vi "Load Becker-Hickl File.vi"(8 "Error In":errorcluster, 11 "File Path Control":path) -> (0 "Error Out":errorcluster, 1 "Measurement Information":T1 {"Measurement FCS Info"."FCS Type" format="%.0b"; "Measurement FCS Info"."FCS Decay Calc" format="%016b"; "Measurement Stop Info"."Flags" format="%016b"}, 2 "Data":sgl[][][](array[numeric]), 4 "TAC Parameters":T5 {"Frequency (Hz)" format="%#.6g"; "TAC Range (s)" format="%.6g"; "TAC Bin (s)" format="%#.6g"}, 5 "Size (in Bytes)":i64, 7 "Load Time (s)":dbl)   [LabVIEW 2021, in "Becker-Hickl Files.lvlib"]
uses:
  Becker-Hickl Files.lvlib
  Time/Time.lvlib
  Becker-Hickl Image Parameters.ctl
  Becker-Hickl TAC Parameters.ctl
  Becker-Hickl Measurement Stop Info.ctl
  Becker-Hickl FCS Measurement Info.ctl
  Becker-Hickl Additional Histogram Measurement Info.ctl
  Becker-Hickl Measurement Information.ctl
  Becker-Hickl File Header Structure.ctl
panel:
  out "Image Parameters":T6
  out "B& H File Header":T7 {"Header Valid" format="%.0x"; "# Data Blocks" format="%.0x"; "Revision" format="%.0b"}
  out "Information String":string
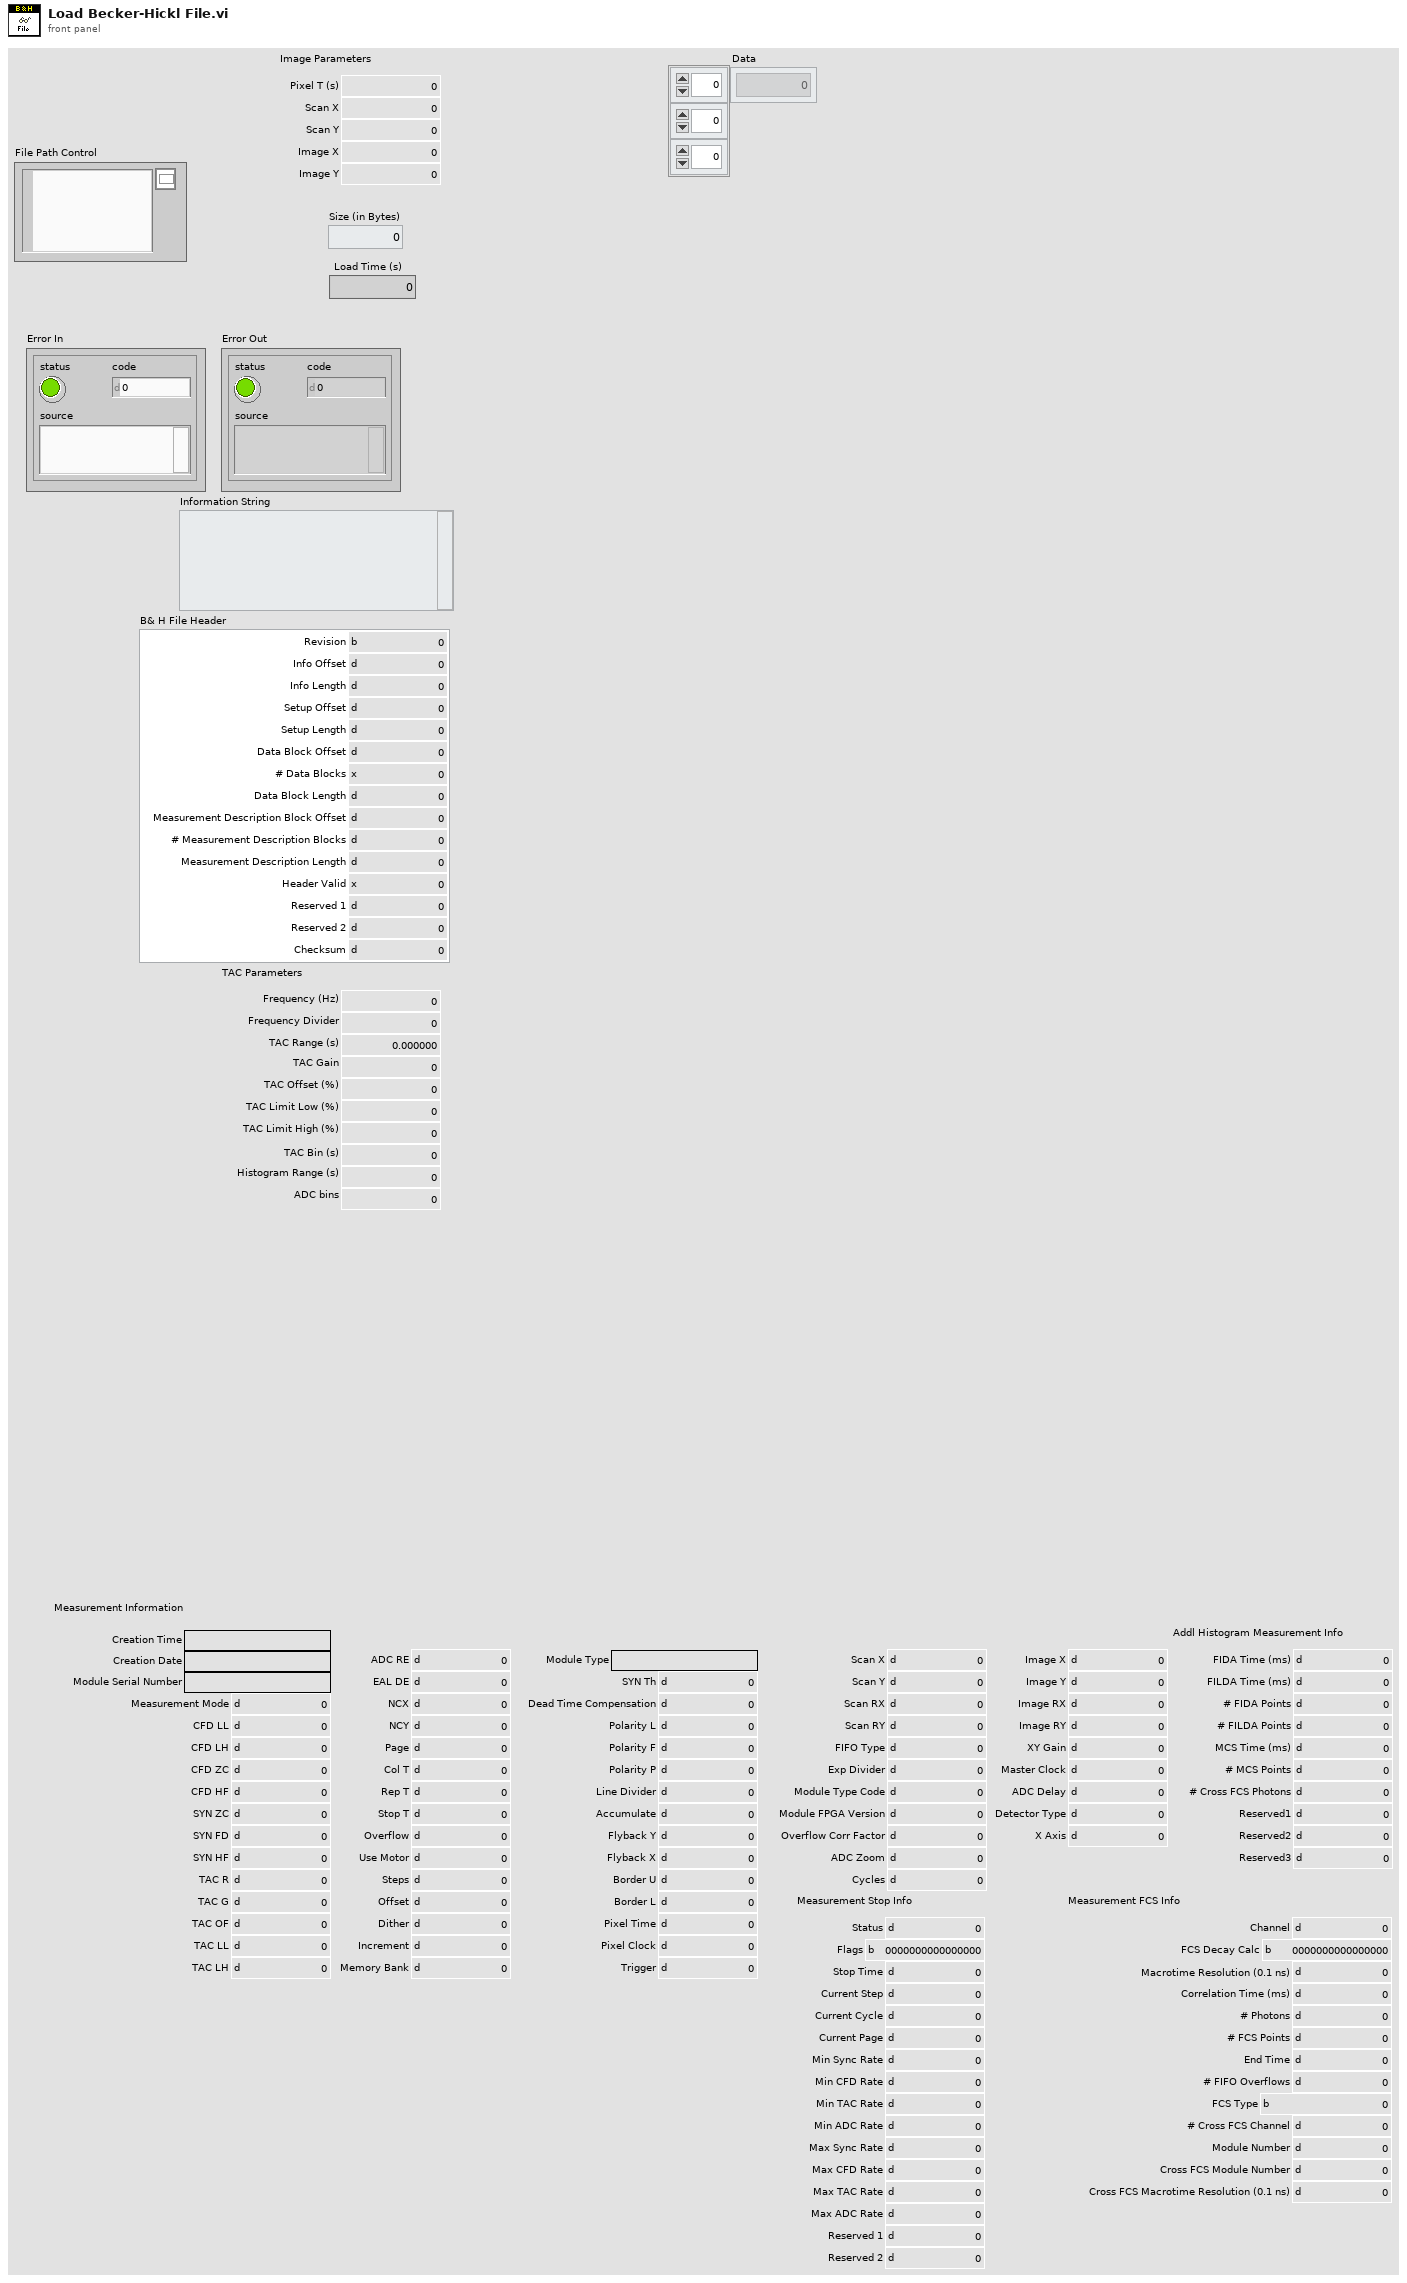
[diagram p1: front panel]
types:
  T1 = typedef "Becker-Hickl Files.lvlib/Becker-Hickl Measurement Information.ctl" = cluster{"Measurement Stop Info":T2, "Measurement FCS Info":T3, "Addl Histogram Measurement Info":T4, "Creation Time":string, "Creation Date":string, "Module Serial Number":string, "Measurement Mode":i16, "CFD LL":sgl, "CFD LH":sgl, "CFD ZC":sgl, "CFD HF":sgl, "SYN ZC":sgl, "SYN FD":i16, "SYN HF":sgl, "TAC R":sgl, "TAC G":i16, "TAC OF":sgl, "TAC LL":sgl, "TAC LH":sgl, "ADC RE":i16, "EAL DE":i16, "NCX":i16, "NCY":i16, "Page":u16, "Col T":sgl, "Rep T":sgl, "Stop T":i16, "Overflow":u8, "Use Motor":i16, "Steps":u16, "Offset":sgl, "Dither":i16, "Increment":i16, "Memory Bank":i16, "Module Type":string, "SYN Th":sgl, "Dead Time Compensation":i16, "Polarity L":i16, "Polarity F":i16, "Polarity P":i16, "Line Divider":i16, "Accumulate":i16, "Flyback Y":i32, "Flyback X":i32, "Border U":i32, "Border L":i32, "Pixel Time":sgl, "Pixel Clock":i16, "Trigger":i16, "Scan X":i32, "Scan Y":i32, "Scan RX":i32, "Scan RY":i32, "FIFO Type":i16, "Exp Divider":i32, "Module Type Code":u16, "Module FPGA Version":u16, "Overflow Corr Factor":sgl, "ADC Zoom":i32, "Cycles":i32, "Image X":i32, "Image Y":i32, "Image RX":i32, "Image RY":i32, "XY Gain":i16, "Master Clock":i16, "ADC Delay":i16, "Detector Type":i16, "X Axis":i16}
  T2 = typedef "Becker-Hickl Files.lvlib/Becker-Hickl Measurement Stop Info.ctl" = cluster{"Status":u16, "Flags":u16, "Stop Time":sgl, "Current Step":i32, "Current Cycle":i32, "Current Page":i32, "Min Sync Rate":sgl, "Min CFD Rate":sgl, "Min TAC Rate":sgl, "Min ADC Rate":sgl, "Max Sync Rate":sgl, "Max CFD Rate":sgl, "Max TAC Rate":sgl, "Max ADC Rate":sgl, "Reserved 1":i32, "Reserved 2":sgl}
  T3 = typedef "Becker-Hickl Files.lvlib/Becker-Hickl FCS Measurement Info.ctl" = cluster{"Channel":u16, "FCS Decay Calc":u16, "Macrotime Resolution (0.1 ns)":u32, "Correlation Time (ms)":sgl, "# Photons":u32, "# FCS Points":i32, "End Time":sgl, "# FIFO Overflows":u16, "FCS Type":u16, "# Cross FCS Channel":u16, "Module Number":u16, "Cross FCS Module Number":u16, "Cross FCS Macrotime Resolution (0.1 ns)":u32}
  T4 = typedef "Becker-Hickl Files.lvlib/Becker-Hickl Additional Histogram Measurement Info.ctl" = cluster{"FIDA Time (ms)":sgl, "FILDA Time (ms)":sgl, "# FIDA Points":i32, "# FILDA Points":i32, "MCS Time (ms)":sgl, "# MCS Points":i32, "# Cross FCS Photons":u32, "Reserved1":i32, "Reserved2":dbl, "Reserved3":dbl}
  T5 = typedef "Becker-Hickl Files.lvlib/Becker-Hickl TAC Parameters.ctl" = cluster{"Frequency (Hz)":dbl, "Frequency Divider":i32, "TAC Range (s)":dbl, "TAC Gain":i32, "TAC Offset (%)":dbl, "TAC Limit Low (%)":dbl, "TAC Limit High (%)":dbl, "TAC Bin (s)":dbl, "ADC bins":i32, "Histogram Range (s)":dbl}
  T6 = typedef "Becker-Hickl Files.lvlib/Becker-Hickl Image Parameters.ctl" = cluster{"Pixel T (s)":dbl, "Scan X":i32, "Scan Y":i32, "Image X":i32, "Image Y":i32}
  T7 = typedef "Becker-Hickl Files.lvlib/Becker-Hickl File Header Structure.ctl" = cluster{"Revision":i16, "Info Offset":i32, "Info Length":i16, "Setup Offset":i32, "Setup Length":i16, "Data Block Offset":i32, "# Data Blocks":i16, "Data Block Length":i32, "Measurement Description Block Offset":i32, "# Measurement Description Blocks":i16, "Measurement Description Length":i16, "Header Valid":u16, "Reserved 1":u32, "Reserved 2":u16, "Checksum":u16}
  T8 = typedef "Becker-Hickl Files.lvlib/Becker-Hickl FLIM Image Sizes.ctl" = cluster{"Image X":i32, "Image Y":i32, "ADC bins":i32}
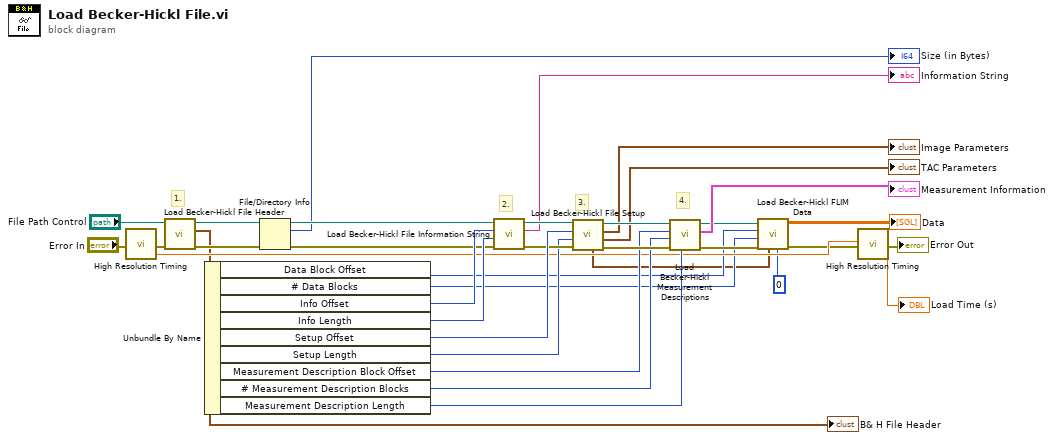
[diagram p0: block diagram]
diagram:
  # "4."
  # "1."
  # "3."
  # "2."
  n1 = call "High Resolution Timing.vi"("Error In"="Error In") -> ("elapsed (relative) seconds"=w15:dbl, "Error Out"=w17:errorcluster)  [unwired: 16 in, 1 out]
  n2 = call "Load Becker-Hickl File Header.vi"("Error In"=w17, "File Path Control"="File Path Control") -> ("Error Out"=w20:errorcluster, "B& H File Header"=w12:T7, "File Path out"=w35:path)  [unwired: 7 in]
  "B& H File Header" <- w12
  n3 = Unbundle By Name(w12) -> ("Data Block Offset"=w4:i32, "# Data Blocks"=w3:i16, "Info Offset"=w32:i32, "Info Length"=w31:i16, "Setup Offset"=w30:i32, "Setup Length"=w27:i16, "Measurement Description Block Offset"=w24:i32, "# Measurement Description Blocks"=w23:i16, "Measurement Description Length"=w22:i16)
  n4 = File/Directory Info(path=w35, error in=w20) -> (path out=w21:path, size=→"Size (in Bytes)":i64, error out=w19:errorcluster)  [unwired: 4 out]
  n5 = call "Load Becker-Hickl File Information String.vi"("Error In"=w19, "Info Length"=w31, "Info Offset"=w32, "File Path in"=w21) -> ("Error Out"=w28:errorcluster, "Information String"=→"Information String":string, "File Path out"=w29:path)  [unwired: 5 in]
  n6 = call "Load Becker-Hickl File Setup.vi"("Error In"=w28, "Setup Length"=w27, "Setup Offset"=w30, "File Path Control"=w29) -> ("Error Out"=w25:errorcluster, "TAC Parameters"=→"TAC Parameters":T5, "Image Parameters"=→"Image Parameters":T6, "File Path out"=w26:path, "Image Sizes"=w2:T8)  [unwired: 3 in]
  n7 = call "Load Becker-Hickl Measurement Descriptions.vi"("Measurement Description Length"=w22, "Error In"=w25, "# Measurement Description Blocks"=w23, "Measurement Description Block Offset"=w24, "File Path Control"=w26) -> ("Error Out"=w8:errorcluster, "Measurement Information"=→"Measurement Information":T1, "File Path"=w5:path)  [unwired: 4 in]
  n8 = call "Load Becker-Hickl FLIM Data.vi"("Data Block Idx"=0, "Image Sizes"=w2, "error in (no error)"=w8, "# Data Blocks"=w3, "Data Block Offset"=w4, "File Path"=w5) -> ("error out"=w7:errorcluster, "Data"=→"Data":sgl[][][])  [unwired: 4 in]
  n9 = call "High Resolution Timing.vi"("relative seconds (NaN)"=w15, "Error In"=w7) -> ("elapsed (relative) seconds"=→"Load Time (s)":dbl, "Error Out"=→"Error Out":errorcluster)  [unwired: 15 in, 1 out]
